vi "heartBeatReadCreate.vi"(8 "error in (no error)":errorcluster, 10 "interface object in":refnum<k20>, 11 "MotorController in":refnum<class "MotorController.lvclass">) -> (0 "error out":errorcluster, 1 "heartbeat object out":refnum<k20>, 2 "interface object out":refnum<k20>, 3 "MotorController out":refnum<class "MotorController.lvclass">)   [LabVIEW 2018, in "MotorController.lvclass"]
uses:
  MotorController.lvclass
  MotorController.lvclass/MotorController.ctl
  <vilib>/CANopenLib/CANOPEN.llb/CANopen Heartbeat Create.vi
  <vilib>/CANopenLib/CANOPEN.llb/CANopen Heartbeat Start.vi
panel:
  out "completion code":u32
  out "description":string
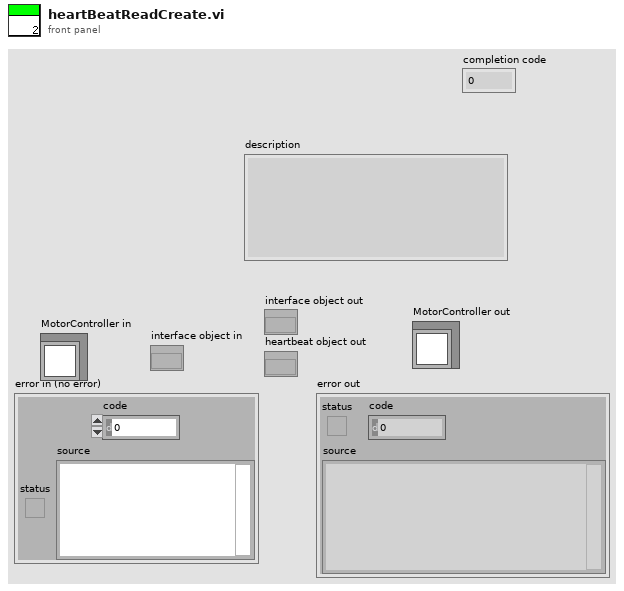
[diagram p1: front panel]
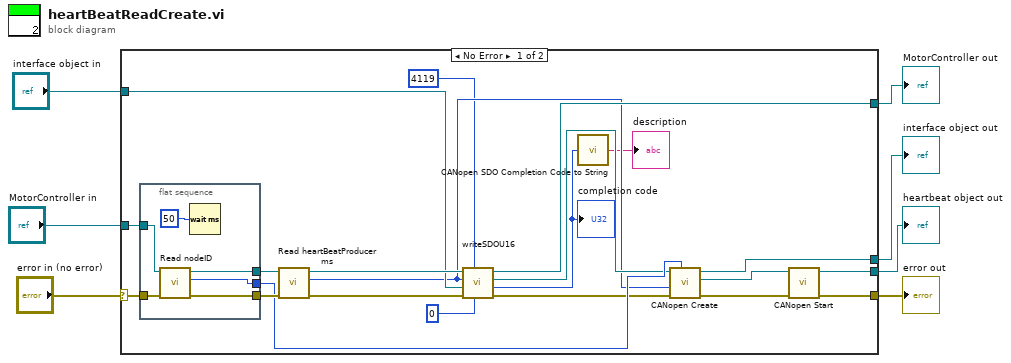
[diagram p0: block diagram]
diagram:
  n1 = case shown="No Error" "error in (no error)" {
    selector: "error in (no error)" -> [w24 w37]
    tunnel: [w20 w37] -> w6
    tunnel: [w18 w36] -> w4
    tunnel: "MotorController in" -> [w25 w36]
    tunnel: "interface object in" -> [w13 w35]
    tunnel: [w21 _] -> w2
    tunnel: [w19 w35] -> w1
    frame No Error {
      n2 = flat-sequence {
        tunnel: [w34] -> w28
        tunnel: [w33] -> w26
        tunnel: w25 -> [w32]
        tunnel: w24 -> [w31]
        tunnel: [w30] -> w23
        frame #0 {
          n3 = call "Read nodeID.vi"("error in (no error)"=w31, "MotorController in"=w32) -> ("error out"=w34:errorcluster, "nodeID"=w30:u8, "MotorController out"=w33:refnum<class "MotorController.lvclass">)  [unwired: 7 in]
          n4 = Wait (ms)(milliseconds to wait=u32 50) -> ()  [unwired: 1 out]
        }
      }
      n5 = call "Read heartBeatProducer ms.vi"("error in (no error)"=w28, "MotorController in"=w26) -> ("error out"=w16:errorcluster, "heartBeatProducer ms"=w11:u16, "MotorController out"=w17:refnum<class "MotorController.lvclass">)  [unwired: 7 in]
      n6 = call "writeSDOU16.vi"("object sub-index (0)"=u8 0, "object index"=u16 4119, "error in (no error)"=w16, "interface object in"=w13, "inputNumber"=w11, "MotorController in"=w17) -> ("error out"=w15:errorcluster, "completion code"=w10:u32, "interface object out"=w12:refnum<k20>, "MotorController out"=w18:refnum<class "MotorController.lvclass">)  [unwired: 2 in]
      "completion code" <- w10
      n7 = call <vilib>:"CANopen SDO Completion Code to String.vi"("SDO completion code"=w10) -> ("description"=→"description":string)
      n8 = call-poly <vilib>:"CANopen Create.vi"("node-ID"=w23, "error in (no error)"=w15, "consumer time [ms]"=w11, "interface object in"=w12) -> ("error out"=w27:errorcluster, "heartbeat object out"=w22:refnum<k20>, "interface object out"=w19:refnum<k20>)  [unwired: 5 in]
      n9 = call-poly <vilib>:"CANopen Start.vi"("error in (no error)"=w27, "heartbeat object in"=w22) -> ("error out"=w20:errorcluster, "heartbeat object out"=w21:refnum<k20>)  [unwired: 8 in]
    }
    frame Error {
    }
  }
  "error out" <- w6
  "MotorController out" <- w4
  "interface object out" <- w1
  "heartbeat object out" <- w2
